vi "配置文件read.vi"(8 "error in (no error)":errorcluster caption="错误输入（无错误）", 9 "configuration file path":path caption="配置文件的路径", 10 "键数组":string[](array[string]), 11 "段":string="应用程序交互") -> (0 "error out":errorcluster caption="错误输出", 2 "section exists?":bool caption="段存在？", 3 "updateconfiguration":cluster{"IP地址":string, "端口号":i32, "软件版本":string}={"IP地址"="27.154.58.30", "端口号"=10050, "软件版本"=""})   [LabVIEW 2016, in "自动更新.lvlib"]
uses:
  <vilib>/Utility/config.llb/Read Key (I32).vi
  <vilib>/Utility/config.llb/Read Key (String).vi
  <vilib>/Utility/config.llb/Write Key (Boolean).vi
  <vilib>/Utility/config.llb/NI_LVConfig.lvlib
  <vilib>/Utility/Data Type/NI_Data Type.lvlib
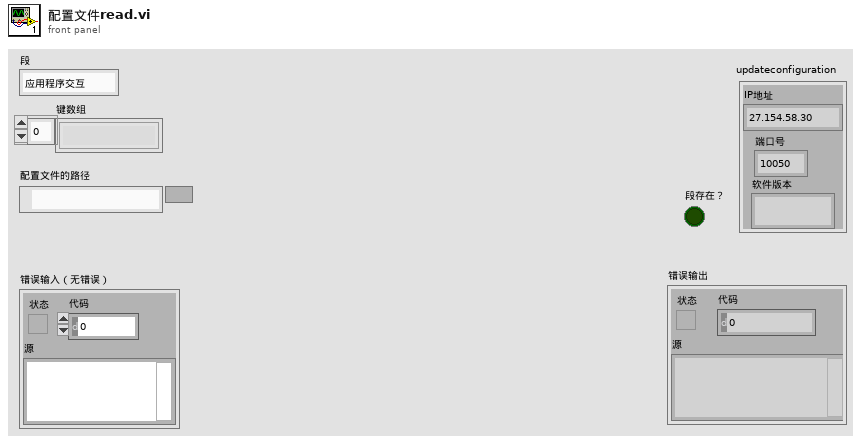
[diagram p1: front panel]
types:
  T1 = typedef "NI_LVConfig.lvlib/Config Data RefNum.ctl" = refnum<k1>
  T2 = typedef "NI_Data Type.lvlib/Data Type.ctl" = enum8{"Invalid Type", "Void", "I8", "I16", "I32", "I64", "U8", "U16", "U32", "U64", "Single Float", "Double Float", "Extended Float", "Single Complex", "Double Complex", "Extended Complex", "Enum U8", "Enum U16", "Enum U32", "Enum U64", "Single Float With Unit", "Double Float With Unit", "Extended Float With Unit", "Single Complex with Unit", "Double Complex with Unit", "Extended Complex with Unit", "Boolean", "String", "Path", "Picture", "Tag", "Array", "Cluster", "Variant", "LV Variant", "Waveform", "Timestamp", "Digital Waveform", "Digital Data", "ExpressData", "Refnum", "External Data", "VI", "Poly VI", "LabVIEW Class Instance", "Fixed Point"}
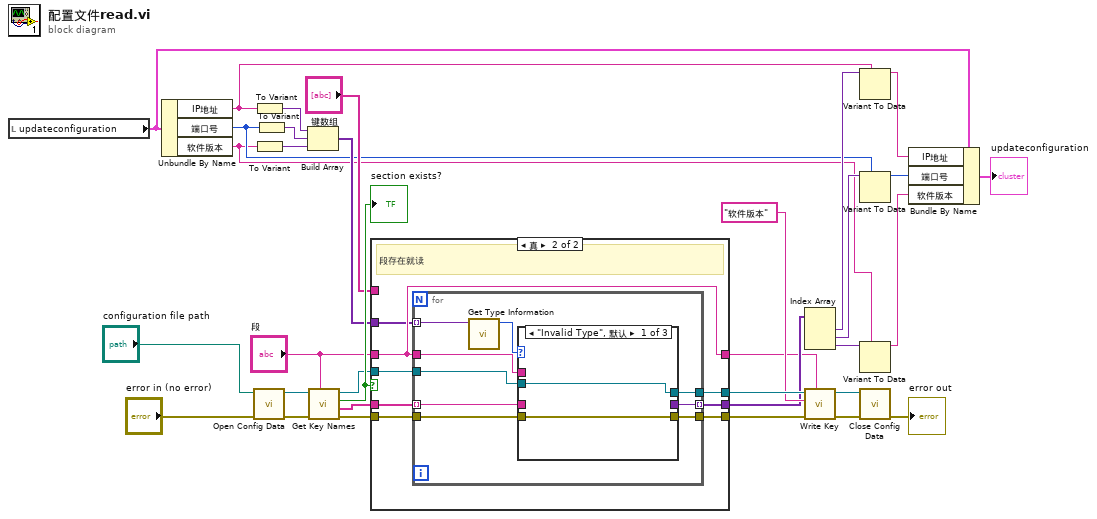
[diagram p0: block diagram]
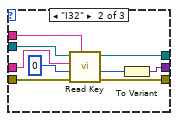
[diagram p3: hidden frame]
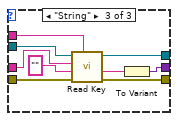
[diagram p4: hidden frame]
diagram:
  n1 = local read "updateconfiguration"() -> (w14:cluster{"IP地址":string, "端口号":i32, "软件版本":string})
  n2 = Unbundle By Name(w14) -> ("IP地址"=w6:string, "端口号"=w5:i32, "软件版本"=w4:string)
  n3 = call <vilib>:"Open Config Data.vi"("error in (no error)"="error in (no error)", "configuration file path"="configuration file path") -> ("error out"=w32:errorcluster, "refnum"=w33:T1)  [unwired: 7 in, 1 out]
  n4 = To Variant(anything=w6) -> (Variant=w13:variant)
  n5 = To Variant(anything=w4) -> (Variant=w11:variant)
  n6 = To Variant(anything=w5) -> (Variant=w12:variant)
  n7 = Build Array(w13, w12, w11) -> (w10:variant[])
  n8 = call <vilib>:"Get Key Names.vi"("section"="段", "error in (no error)"=w32, "refnum"=w33) -> ("error out"=w29:errorcluster, "key names"=w28:string[], "section exists?"=w31:bool, "refnum out"=w30:T1)  [unwired: 5 in]
  "section exists?" <- w31
  n9 = case shown="真" w31 {
    tunnel: w30 -> [w35 w43]
    tunnel: w29 -> [w34 w42]
    tunnel: w28 -> [_ w44]
    tunnel: "段" -> [w36 w38]
    tunnel: [_ w41] -> w21
    tunnel: [w35 w40] -> w27
    tunnel: [w34 w39] -> w24
    tunnel: [w36 w38] -> w20
    tunnel: "键数组" -> [_ _]
    tunnel: w10 -> [_ w37]
    frame False {
      # "段不存在就赋初值"
    }
    frame True {
      # "段存在就读"
      n10 = for {
        tunnel: w44 -> [w48] mode=indexing
        tunnel: w43 -> [w50]
        tunnel: w42 -> [w47]
        tunnel: w38 -> [w51]
        tunnel: [w45] -> w41 mode=indexing
        tunnel: [w49] -> w40
        tunnel: [w46] -> w39
        tunnel: w37 -> [w52] mode=indexing
        n11 = call <vilib>:"Get Type Information.vi"("Variant"=w52) -> ("Type"=w53:T2)  [unwired: 6 in, 4 out]
        n12 = case shown="\"Invalid Type\", 默认" w53 {
          tunnel: w51 -> [_ w63 w72]
          tunnel: w50 -> [w55 w61 w71]
          tunnel: [w55 w60 w70] -> w49
          tunnel: w48 -> [_ w62 w69]
          tunnel: w47 -> [w54 w58 w68]
          tunnel: [w54 w57 w67] -> w46
          tunnel: [_ w56 w65] -> w45
          frame "Invalid Type", Default {
          }
          frame "I32" {
            n13 = call-poly <vilib>:"Read Key.vi"("section"=w63, "error in (no error)"=w58, "default value"=0, "key"=w62, "refnum"=w61) -> ("error out"=w57:errorcluster, "value"=w59:i32, "refnum out"=w60:T1)  [unwired: 3 in, 1 out]
            n14 = To Variant(anything=w59) -> (Variant=w56:variant)
          }
          frame "String" {
            n15 = call-poly <vilib>:"Read Key.vi"("section"=w72, "error in (no error)"=w68, "default value"="", "key"=w69, "refnum"=w71) -> ("error out"=w67:errorcluster, "value"=w66:string, "refnum out"=w70:T1)  [unwired: 3 in, 1 out]
            n16 = To Variant(anything=w66) -> (Variant=w65:variant)
          }
        }
      }
    }
  }
  n17 = Index Array(array=w21) -> (element #1=w9:variant, element #2=w8:variant, element #3=w7:variant)  [unwired: 3 in]
  n18 = call-poly <vilib>:"Write Key.vi"("section"=w20, "error in (no error)"=w24, "key"="软件版本", "refnum"=w27) -> ("error out"=w22:errorcluster, "refnum out"=w23:T1)  [unwired: 5 in, 1 out]
  n19 = Variant To Data(type=w6, Variant=w9) -> (data=w3:string)  [unwired: 1 in, 1 out]
  n20 = Variant To Data(type=w5, Variant=w8) -> (data=w2:i32)  [unwired: 1 in, 1 out]
  n21 = Variant To Data(type=w4, Variant=w7) -> (data=w1:string)  [unwired: 1 in, 1 out]
  n22 = call <vilib>:"Close Config Data.vi"("error in (no error)"=w22, "refnum"=w23) -> ("error out"=→"error out":errorcluster)  [unwired: 8 in, 1 out]
  n23 = Bundle By Name(cluster=w14, "IP地址"=w3, "端口号"=w2, "软件版本"=w1) -> (→"updateconfiguration":cluster{"IP地址":string, "端口号":i32, "软件版本":string})
